vi "Service Location FGV.vi"(8 "error in":errorcluster, 10 "Resolve Service Request":T2, 11 "Action":T1) -> (0 "error out":errorcluster, 3 "Service Location":T3)   [LabVIEW 2020, in "gRPC Utilities.lvlib"]
uses:
  gRPC Utilities.lvlib
  MeasurementLink Discovery Client/RPC Messages/ni_measurementlink_discovery_v1_ServiceLocation.ctl
  MeasurementLink Discovery Client/RPC Messages/ni_measurementlink_discovery_v1_ResolveServiceRequest.ctl
  TypeDefs/Service Location FGV Action.ctl
  <vilib>/Utility/miscctls.llb/LVMapReplaceAction.ctl
  GrpcClientPool/FGV Action.ctl
  MeasurementLink Discovery Client/MeasurementLink Discovery Client.lvlib
  GrpcClientPool/GrpcClientPool.lvclass
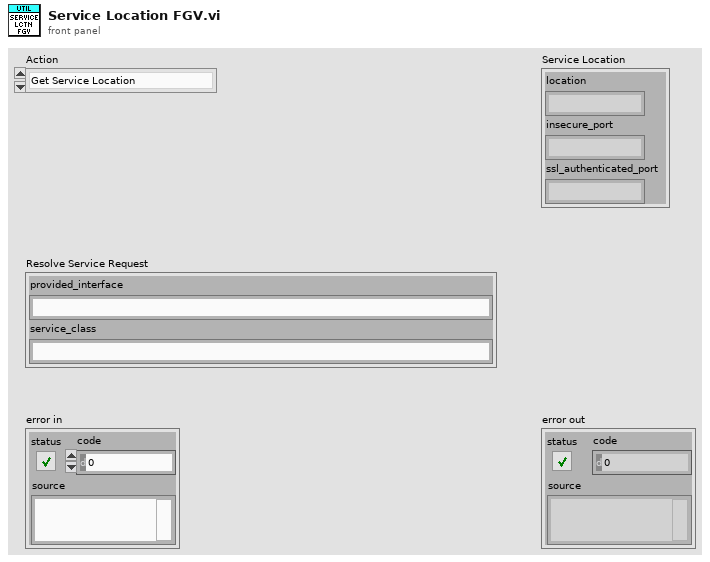
[diagram p1: front panel]
types:
  T1 = typedef "gRPC Utilities.lvlib/Service Location FGV Action.ctl" = enum16{"Get Service Location", "Clear Cache"}
  T2 = typedef "MeasurementLink Discovery Client.lvlib/ni_measurementlink_discovery_v1_ResolveServiceRequest.ctl" = cluster{"provided_interface":string, "service_class":string}
  T3 = typedef "MeasurementLink Discovery Client.lvlib/ni_measurementlink_discovery_v1_ServiceLocation.ctl" = cluster{"location":string, "insecure_port":string, "ssl_authenticated_port":string}
  T4 = typedef "LVMapReplaceAction.ctl" = enum32{"Modify Entry only if found", "Add or Modify Entry", "Delete Entry"}
  T5 = typedef "gRPC Utilities.lvlib/GrpcClientPool.lvclass/FGV Action.ctl" = enum16{"Get Discovery Client", "Get Session Client", "Get Pinmap Client", "Destroy Clients"}
  T6 = typedef "grpc-lvsupport-release.lvlib/grpcId.ctl" = u64
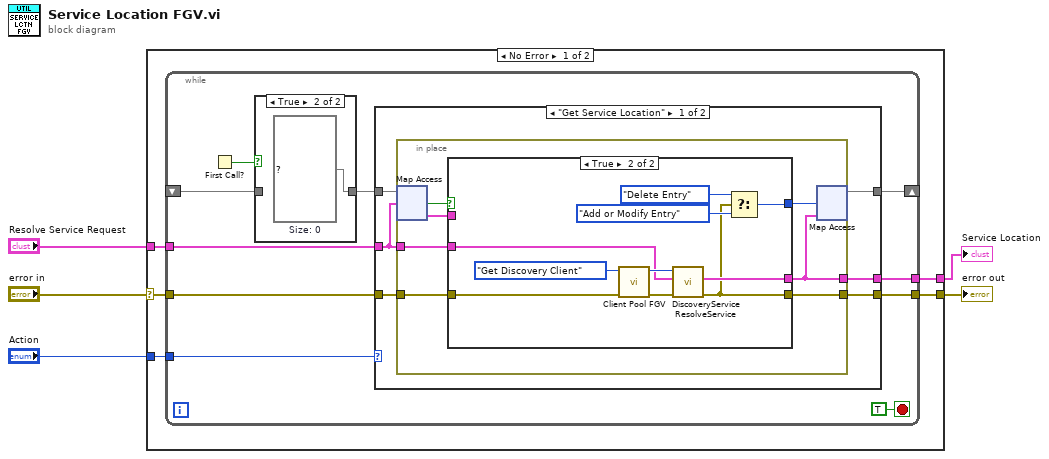
[diagram p0: block diagram]
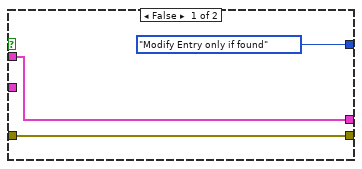
[diagram p3: hidden frame]
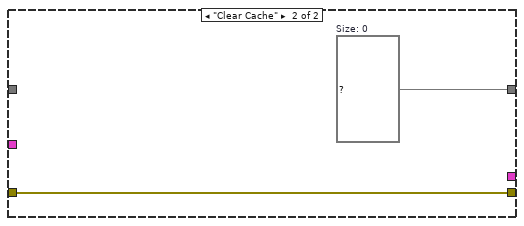
[diagram p4: hidden frame]
diagram:
  n1 = case shown="No Error" "error in" {
    selector: "error in" -> [w10 w51]
    tunnel: [w7 w51] -> w2
    tunnel: [w9 _] -> w5
    tunnel: "Resolve Service Request" -> [w8 _]
    tunnel: "Action" -> [w6 _]
    frame No Error {
      n2 = while {
        shift-right: [w17] -> _
        shift-left: _ -> [w14]
        tunnel: w10 -> [w12]
        tunnel: [w19] -> w9
        tunnel: w8 -> [w18]
        tunnel: [w16] -> w7
        tunnel: w6 -> [w15]
        stop <- TRUE stop-if-true
        n3 = First Call?() -> (First Call?: T/F=w11:bool)
        n4 = case shown="True" w11 {
          tunnel: w14 -> [w21 _]
          tunnel: [w21 w22] -> w13
          frame False {
          }
          frame True {
            w22 = map{T2, T3} {}  # Size: 0
          }
        }
        n5 = case shown="\"Get Service Location\"" w15 {
          tunnel: w13 -> [w25 _]
          tunnel: [w28 _] -> w19
          tunnel: w18 -> [w23 _]
          tunnel: w12 -> [w26 w50]
          tunnel: [w24 w49] -> w17
          tunnel: [w27 w50] -> w16
          frame "Get Service Location" {
            n6 = in-place {
              in-place-border: w26 -> [w35]
              in-place-border: [w31] -> w28
              in-place-border: [w34] -> w27
              in-place-border: w23 -> [w29]
              n7 = in-place-map #1(w25, w23) -> (w32:T3, w33:bool)  [unwired: 1 in]
              n8 = case shown="True" w33 {
                tunnel: w35 -> [w38 w47]
                tunnel: [w38 w40] -> w34
                tunnel: w32 -> [w37 _]
                tunnel: [w37 w44] -> w31
                tunnel: [LVMapReplaceAction."Modify Entry only if found" ("action") w42] -> w30
                tunnel: w29 -> [_ w39]
                frame False {
                }
                frame True {
                  n9 = call "Client Pool FGV.vi"("error in (no error)"=w47, "Action"=FGV_Action."Get Discovery Client") -> ("error out"=w46:errorcluster, "grpc client id"=w45:T6)  [unwired: 8 in]
                  n10 = call "DiscoveryService ResolveService.vi"("error in"=w46, "Request Data"=w39, "gRPC ID"=w45) -> ("error out"=w40:errorcluster, "Response Data"=w44:T3)  [unwired: 6 in, 1 out]
                  n11 = Select(t=LVMapReplaceAction."Delete Entry", s=w40, f=LVMapReplaceAction."Add or Modify Entry" ("action")) -> (s? t:f=w42:T4)
                }
              }
              n12 = in-place-map #1(w31, w30) -> (w24:map{T2, T3})  [unwired: 2 out]
            }
          }
          frame "Clear Cache" {
            w49 = map{T2, T3} {}  # Size: 0
          }
        }
      }
    }
    frame Error {
    }
  }
  "Service Location" <- w5
  "error out" <- w2
